vi "DAQ 1SDI v07.vi"() -> ()   [LabVIEW 2013]
uses:
  Strict Type Defs/type_meas_enum.ctl
  <instrlib>/niScope/Controls/niScope vertical coupling.ctl
panel:
  in  "stop":bool
  out "Loop count":i32=237879
  in  "Monitors":enum32{"Monitors On", "Monitors Off"}(tab)
  out "covariance HD 1 & 2":dbl(graph)=-0.000466554199747969
  out "Conditional variance HD 1|3":dbl(graph)=0.016266525893794365
  out "Conditional variance HD 2|3":dbl(graph)=0.014702240762452789
  out "covariance HD 2 & 3":dbl(graph)=-0.0010436947745436462
  in  "Settings":enum32{"Settings and Record", "Under the hood"}(tab)=enum."Under the hood"
  in  "Knob":u32(knob)=43 scale=0.0..250.0
  in  "Number of monitor samples":i32=30000 format="%.0p"
  in  "File location":path=path "C:/ni-rt/LabVIEW Data/Aug07/LossHetero/01dB107"
  in  "Type of measurement":T1=enum."electronic"
  in  "File root name":string="Real_01dB"
  in  "Number of samples save":i32=2000000 format="%.0p"
  in  "reset sn":bool
  in  "Shot noise start":bool
  in  "Additional text":string="OPA 1 optical power set to 15mV on HD A.\nOPA 2 optical power set to 15mV on HD B.\nLocal oscillator is set to 5V on HD.\nParametric gain set to 15 for OPA 1.\nParametric gain set to 15 for OPA 2.\nVertical range set to 0.5V for both channels.\nSample rate set to 14MS/s.\nMax input freq set to 7MHz.\nVisibility between OPA 1 & OPA 2 = 99.4\nVisibility between OPA 1 & L.O.1 = 98.8\nVisibility between OPA 1 & L.O. 2 = 98.45\nVisibility between OPA 1 & L.O. 3 = 99.0\nBoth squeezers expected to produce -6.5dB/10dB.\nLoss on EPR B =0.23% (0.1dB)  \n"
  in  "Record":bool
  in  "Number of Files":i32=3
  out "File count":i32=2
  in  "Run":string="4"
  out "Cluster":T2={"Actual samples acquired ch 1"=2000000, "Actual samples acquired ch 0"=2000000, "Actual samples acquired ch 2"=2000000}
  in  "Channel Parms":T4={"Input impedance (Ohms)"=2, "Maximum input frequency (Hz)"=7000000.0, "vertical coupling"=1, "Probe attenuation"=1.0, "Vertical range (V)"=0.5, "Vertical offset"=0.0, "channel enabled"=TRUE} {"Input impedance (Ohms)" items=["1 mega ohm"=0, "50 ohms"=2]; "Maximum input frequency (Hz)" format="%#_6p"; "vertical coupling" items=["AC", "DC", "Ground"]}
  in  "IIR filter specifications":T5={"Topology"=enum."Butterworth", "Type"=enum."Bandpass", "Order"=6, "Lower Fc"=2900000.0, "Upper Fc"=3100000.0, "PB Ripple"=1.0, "SB Attenuation"=60.0} {"PB Ripple" format="%0.2f"; "SB Attenuation" format="%0.2f"; "Lower Fc" format="%0.2p"; "Upper Fc" format="%0.2p"}
  out "error out":errorcluster caption="error out final"
  in  "max time (s)":dbl=10.0 caption="Time to run (s)"
  in  "Reference position":dbl(slide)=50.0 scale=0.0..100.0
  in  "Minimum sample rate (S/s)":dbl=14000000.0 format="%#_6p"
  out "Video bandwidth (Hz)":dbl=7.0
  in  "DAQ Cards":T6={"DAQ Card 1"="Dev2", "DAQ Card 2"="Dev3"}
  # "Variance won't be displayed until shot noise is taken"
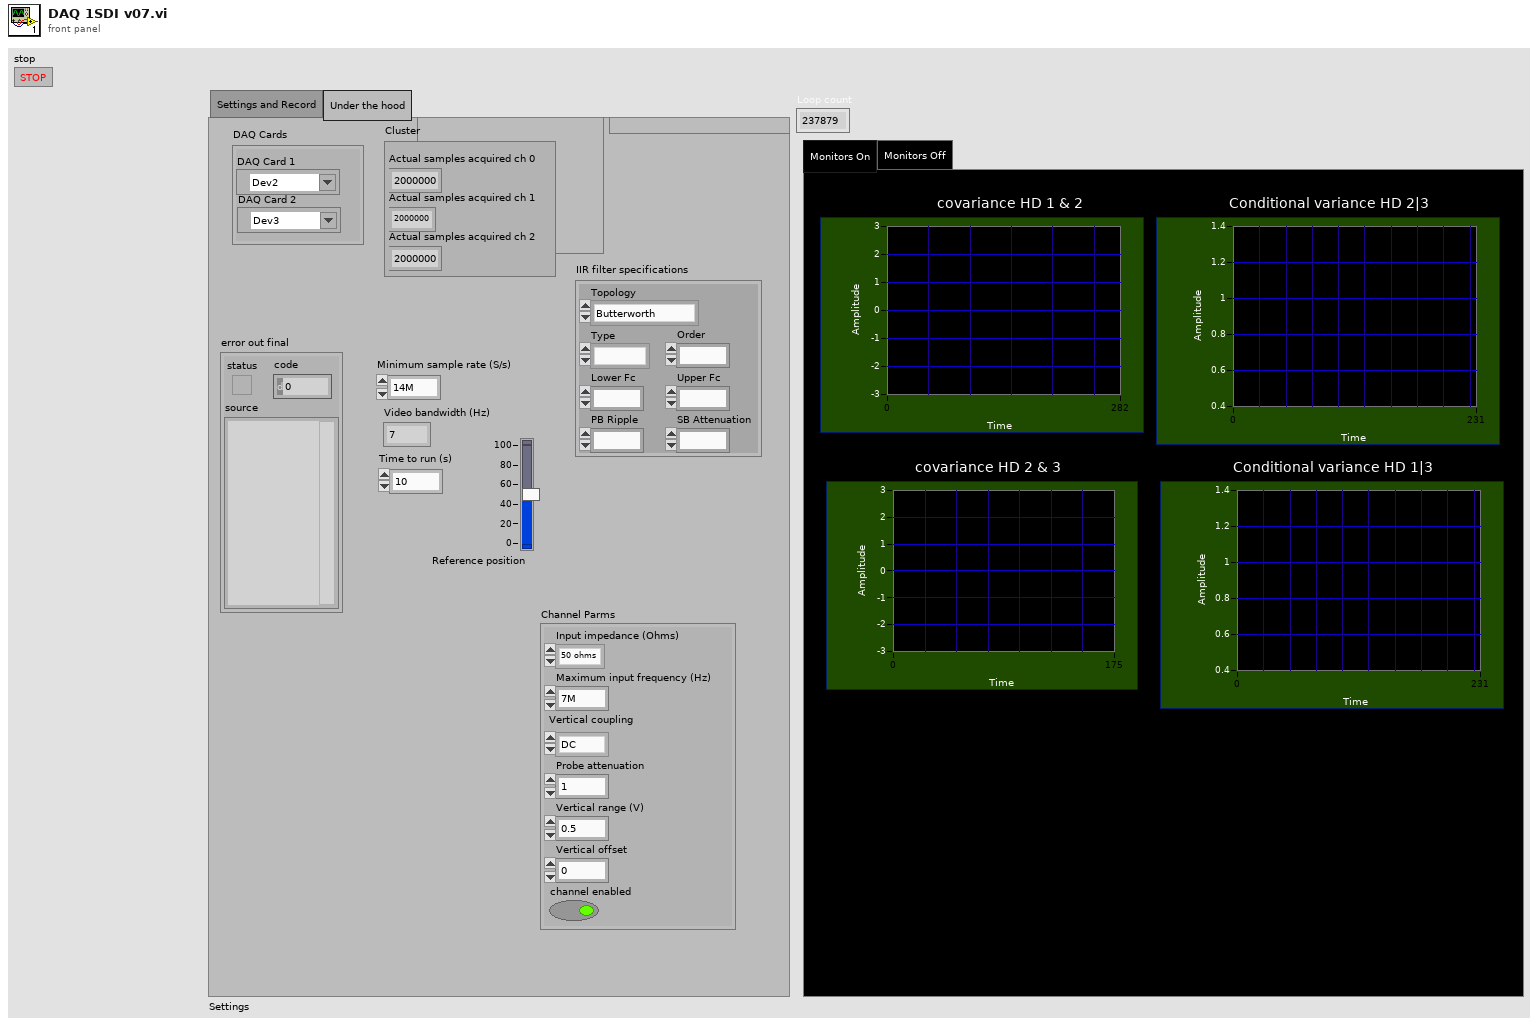
[diagram p1: front panel]
types:
  T1 = typedef "type_meas_enum.ctl" = enum16{"shot", "x", "p", "electronic"}
  T2 = cluster{"Actual samples acquired ch 1":i32, "Actual samples acquired ch 0":i32, "Actual samples acquired ch 2":i32}
  T3 = typedef "niScope vertical coupling.ctl" = i32
  T4 = cluster{"Input impedance (Ohms)":u32, "Maximum input frequency (Hz)":dbl, "vertical coupling":T3, "Probe attenuation":dbl, "Vertical range (V)":dbl, "Vertical offset":dbl, "channel enabled":bool}
  T5 = cluster{"Topology":enum16{"Off", "Butterworth", "Chebyshev", "Inverse Chebyshev", "Elliptic", "Bessel"}, "Type":enum16{"Lowpass", "Highpass", "Bandpass", "Bandstop"}, "Order":i32, "Lower Fc":dbl, "Upper Fc":dbl, "PB Ripple":dbl, "SB Attenuation":dbl}
  T6 = cluster{"DAQ Card 1":refnum<k15>, "DAQ Card 2":refnum<k15>}
  T7 = cluster{"instrument handle":refnum<k15>, "instrument handle":refnum<k15>}
  T8 = cluster{"instrument handle out 0":refnum<k15>, "instrument handle out 1":refnum<k15>}
  T9 = cluster{"actualSamples":i32, "actualSamples":i32, "actualSamples":i32}
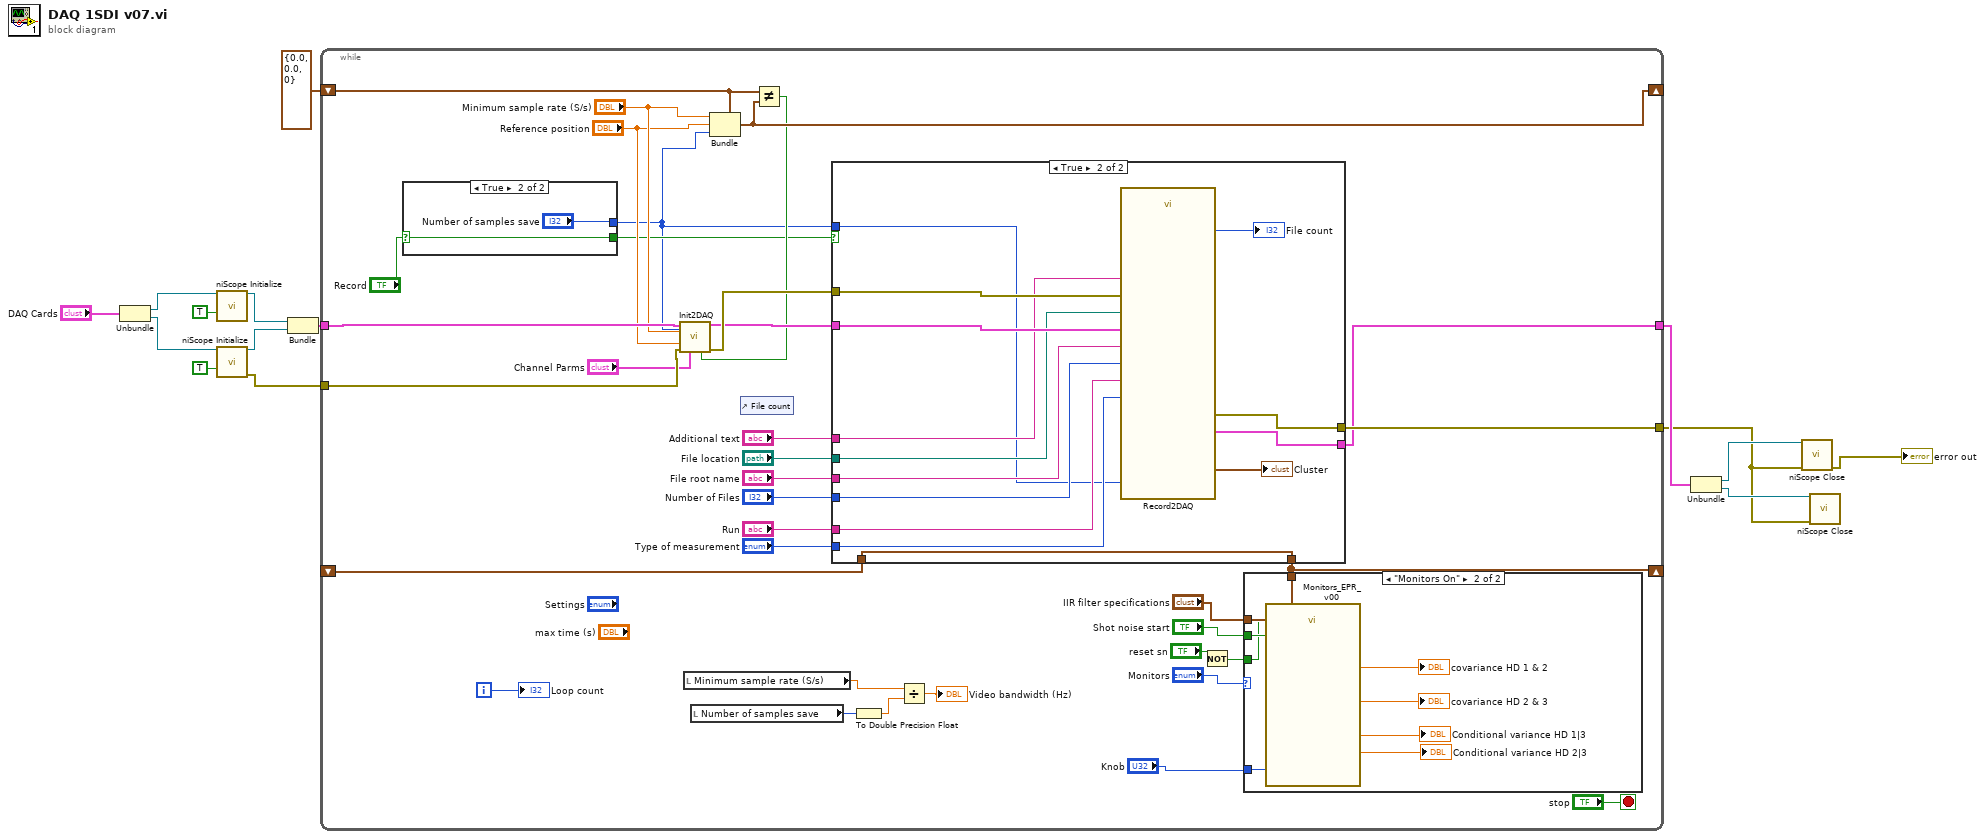
[diagram p0: block diagram]
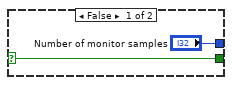
[diagram p2: hidden frame]
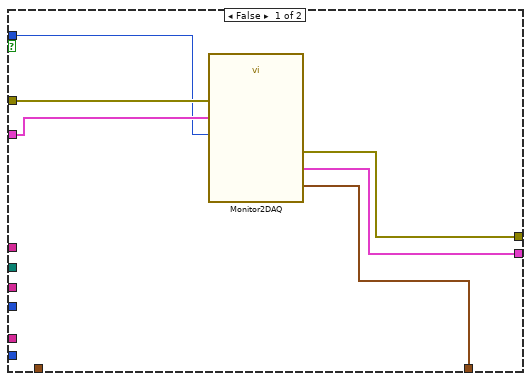
[diagram p4: hidden frame]
diagram:
  n1 = Unbundle("DAQ Cards") -> ("DAQ Card 1"=w7:refnum<k15>, "DAQ Card 2"=w6:refnum<k15>)
  n2 = call <instrlib>:"niScope Initialize.vi"("resource name"=w7, "reset device"=TRUE) -> ("instrument handle"=w4:refnum<k15>)  [unwired: 12 in, 1 out]
  n3 = call <instrlib>:"niScope Initialize.vi"("resource name"=w6, "reset device"=TRUE) -> ("instrument handle"=w3:refnum<k15>, "error out"=w5:errorcluster)  [unwired: 12 in]
  n4 = Bundle("instrument handle"=w4, "instrument handle"=w3) -> (w2:T7)  [unwired: 1 in]
  n5 = while {
    tunnel: [w44] -> w11
    tunnel: w5 -> [w30]
    shift-right: [w25] -> _
    shift-left: cluster{dbl, dbl, i32} {0.0, 0.0, 0} -> [w26]
    shift-right: [w20] -> _
    shift-left: _ -> [w19]
    tunnel: w2 -> [w31]
    tunnel: [w33] -> w15
    i -> [w46]
    stop <- "stop" stop-if-true
    n6 = case shown="True" "Record" {
      selector: "Record" -> [w52 w54]
      tunnel: ["Number of monitor samples" "Number of samples save"] -> w16
      tunnel: [w52 w54] -> w21
      frame False {
      }
      frame True {
      }
    }
    n7 = local read "Minimum sample rate (S/s)"() -> (w34:dbl)
    n8 = local read "Number of samples save"() -> (w36:i32)
    n9 = Bundle(cluster=w26, "Minimum sample rate (S/s)", "Reference position", w16) -> (w25:cluster{dbl, dbl, i32})
    n10 = control-ref of="File count"() -> ()  [unwired: 1 out]
    n11 = Not Equal?(x=w26, y=w25) -> (x != y?=w24:bool)
    n12 = call "Init2DAQ.vi"("resource names"=w31, "min record length"=w16, "min sample rate"="Minimum sample rate (S/s)", "reference position"="Reference position", "error in"=w30, "channel parms"="Channel Parms", "Ch param"=w24) -> ("instrument out"=w32:T8, "error out"=w50:errorcluster)  [unwired: 7 in]
    n13 = case shown="True" w21 {
      tunnel: w32 -> [w68 w83]
      tunnel: w50 -> [w69 w82]
      tunnel: [w67 w81] -> w44
      tunnel: "Additional text" -> [_ w80]
      tunnel: "File location" -> [_ w79]
      tunnel: "File root name" -> [_ w78]
      tunnel: "Number of Files" -> [_ w77]
      tunnel: "Run" -> [_ w76]
      tunnel: "Type of measurement" -> [_ w75]
      tunnel: [w66 w71] -> w20
      tunnel: [w65 w72] -> w33
      tunnel: w19 -> [_ w71]
      tunnel: w16 -> [w64 w70]
      frame False {
        n14 = call "Monitor2DAQ.vi"("instrument in"=w68, "error in"=w69, "numSamples"=w64) -> ("instrument out"=w65:T8, "wfm"=w66:waveform(dbl)[], "error out"=w67:errorcluster)  [unwired: 10 in]
      }
      frame True {
        n15 = call "Record2DAQ.vi"("instrument in"=w83, "Additional text"=w80, "numSamples"=w70, "File location"=w79, "Type of\nmeasurement"=w75, "Name root"=w78, "error in"=w82, "Run"=w76, "number of files"=w77) -> ("output cluster"=→"Cluster":T9, "instrument out"=w72:T8, "File count"=→"File count":i32, "error out"=w81:errorcluster)  [unwired: 2 in, 1 out]
      }
    }
    n16 = To Double Precision Float(number=w36) -> (double precision float=w35:dbl)
    n17 = Divide(x=w34, y=w35) -> (x/y=→"Video bandwidth (Hz)":dbl)
    n18 = Not(x="reset sn") -> (.not. x?=w29:bool)
    n19 = case shown="\"Monitors On\"" "Monitors" {
      tunnel: "Shot noise start" -> [_ w63]
      tunnel: "IIR filter specifications" -> [_ w62]
      tunnel: w29 -> [_ w61]
      tunnel: w20 -> [_ w60]
      tunnel: "Knob" -> [_ w55]
      frame "Monitors Off" {
      }
      frame "Monitors On" {
        n20 = call "Monitors_EPR_v00.vi"("IIR filter specifications"=w62, "Wait(mSec)"=w55, "reset SN"=w61, "Shot noise start"=w63, "wfm"=w60) -> ("covariance B01"=→"covariance HD 1 & 2":dbl, "covariance B1A"=→"covariance HD 2 & 3":dbl, "conditional variance B1|A"=→"Conditional variance HD 2|3":dbl, "conditional variance B0|A"=→"Conditional variance HD 1|3":dbl)  [unwired: 5 in, 2 out]
      }
    }
    "Loop count" <- w46
  }
  n21 = Unbundle(w15) -> ("instrument handle out 0"=w14:refnum<k15>, "instrument handle out 1"=w13:refnum<k15>)
  n22 = call <instrlib>:"niScope Close.vi"("instrument handle"=w14, "error in"=w11) -> ("error out"=→"error out":errorcluster)  [unwired: 13 in]
  n23 = call <instrlib>:"niScope Close.vi"("instrument handle"=w13, "error in"=w11) -> ()  [unwired: 13 in, 1 out]
